vi "SQL插入命令.vi"(9 "插入数值":string[](array[string]), 10 "段名":string[](array[string]), 11 "table":string) -> (3 "SQL插入命令":string)   [LabVIEW 2016, in "数据传输系统-03.lvlib"]
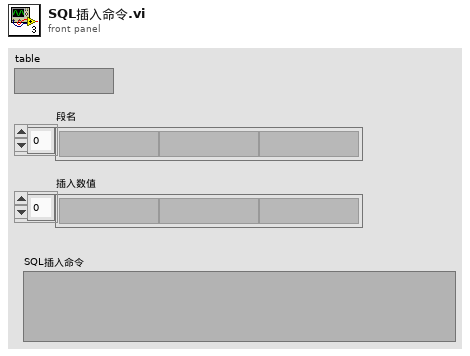
[diagram p1: front panel]
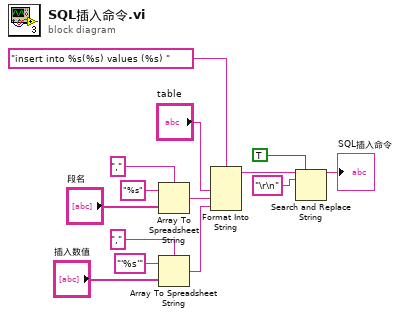
[diagram p0: block diagram]
diagram:
  n1 = Array To Spreadsheet String(delimiter (Tab)="," ("分隔符(Tab)"), array="段名", 3:"%s" ("格式字符串")) -> (spreadsheet string=w5:string)
  n2 = Array To Spreadsheet String(delimiter (Tab)="," ("分隔符(Tab)"), array="插入数值", 3:"'%s'" ("格式字符串")) -> (spreadsheet string=w9:string)
  n3 = Format Into String(format string="insert into %s(%s) values (%s) " ("格式字符串"), "table", w5, w9) -> (resulting string=w10:string)  [unwired: 2 in, 1 out]
  n4 = Search and Replace String(replace all?=TRUE ("替换全部？(F)"), input string=w10, search string="\r\n" ("搜索字符串")) -> (result string=→"SQL插入命令":string)  [unwired: 5 in, 3 out]
